vi "TurnToAngle.vi"() -> ()   [LabVIEW 2017]
uses:
  Framework/Robot Global Data.vi
panel:
  in  "NoWait":bool
  in  "Angle":dbl
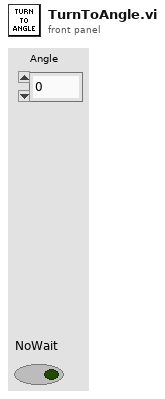
[diagram p1: front panel]
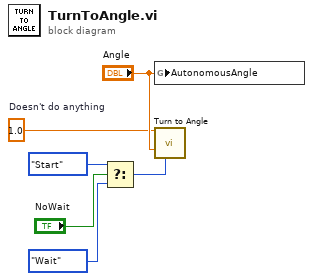
[diagram p0: block diagram]
diagram:
  w5 = 1.0  # Doesn't do anything
  n1 = Select(t=enum16{"Start", "Wait"}."Start", s="NoWait", f=enum16{"Start", "Wait"}."Wait" ("Synchronication")) -> (s? t:f=w1:enum16{"Start", "Wait"})
  n2 = global write "Robot Global Data.vi" "AutonomousAngle"("Angle") -> ()
  n3 = call "Turn to Angle.vi"("Speed"=w5, "Target Angle"="Angle", "Synchronication"=w1) -> ()  [unwired: 12 in, 1 out]
